vi "SecondaryJoystickButtonMapping.vi"(0 "Secondary joystick buttons":bool[](array[boolean])) -> (4 "SecondaryJoystickButtons":T1, 14 "Secondary joystick buttons indicator":bool[](array[boolean]))   [LabVIEW 2018]
uses:
  Controls/SecondaryJoystickButtons.ctl
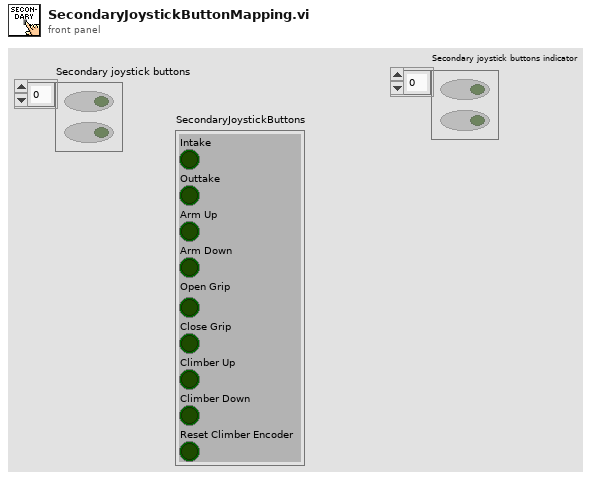
[diagram p1: front panel]
types:
  T1 = typedef "SecondaryJoystickButtons.ctl" = cluster{"Intake":bool, "Outtake":bool, "Arm Up":bool, "Arm Down":bool, "Open Grip":bool, "Close Grip":bool, "Climber Up":bool, "Climber Down":bool, "Reset Climber Encoder":bool}
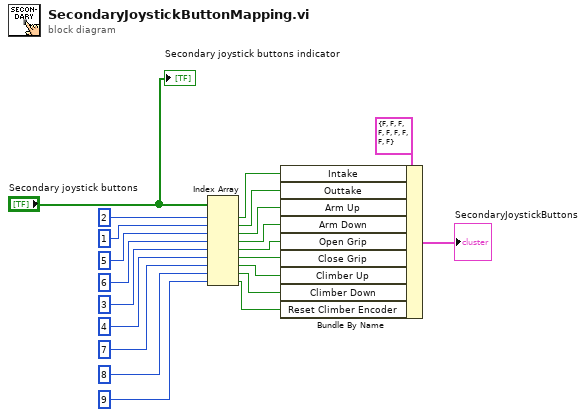
[diagram p0: block diagram]
diagram:
  n1 = Index Array(array="Secondary joystick buttons", index #1=2 ("index"), index #2=1 ("index"), index #3=5 ("index"), index #4=6 ("index"), index #5=3 ("index"), index #6=4 ("index"), index #7=7 ("index"), index #8=8 ("index"), index #9=9 ("index")) -> (element #1=w12:bool, element #2=w11:bool, element #3=w10:bool, element #4=w9:bool, element #5=w8:bool, element #6=w7:bool, element #7=w6:bool, element #8=w4:bool, element #9=w2:bool)
  n2 = Bundle By Name(cluster=T1 {"Intake"=FALSE, "Outtake"=FALSE, "Arm Up"=FALSE, "Arm Down"=FALSE, "Open Grip"=FALSE, "Close Grip"=FALSE, "Climber Up"=FALSE, "Climber Down"=FALSE, "Reset Climber Encoder"=FALSE} ("SecondaryJoystickButtons"), "Intake"=w12, "Outtake"=w11, "Arm Up"=w10, "Arm Down"=w9, "Open Grip"=w8, "Close Grip"=w7, "Climber Up"=w6, "Climber Down"=w4, "Reset Climber Encoder"=w2) -> (→"SecondaryJoystickButtons":T1)
  "Secondary joystick buttons indicator" <- "Secondary joystick buttons"
